vi "Reset SigGen.vi"(8 "error in (no error)":errorcluster, 11 "VISA Refnum in":refnum<visa-resource-name>) -> (0 "error out":errorcluster, 3 "VISA Refnum out":refnum<visa-resource-name>)   [LabVIEW 2015]
uses:
  <instrlib>/Agilent PSG MXG Series/Agilent PSG MXG Series.lvlib
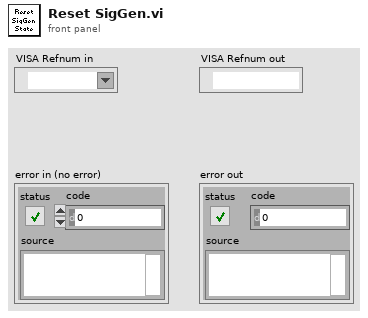
[diagram p1: front panel]
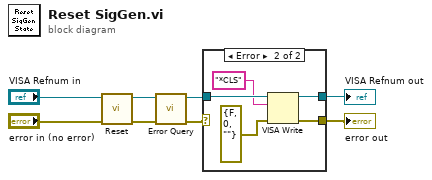
[diagram p0: block diagram]
diagram:
  n1 = call <instrlib>:"Reset.vi"("error in (no error)"="error in (no error)", "VISA resource name"="VISA Refnum in") -> ("error out"=w6:errorcluster, "VISA resource name out"=w5:refnum<visa-resource-name>)  [unwired: 8 in]
  n2 = call <instrlib>:"Error Query.vi"("error in (no error)"=w6, "VISA resource name"=w5) -> ("error out"=w3:errorcluster, "VISA resource name out"=w4:refnum<visa-resource-name>)  [unwired: 6 in, 2 out]
  n3 = case shown="Error" w3 {
    selector: w3 -> [w10 _]
    tunnel: [w9 w15] -> w1
    tunnel: w4 -> [w9 w14]
    tunnel: [w10 w13] -> w2
    frame No Error {
    }
    frame Error {
      n4 = VISA Write(VISA resource name=w14, write buffer="*CLS", error in (no error)=errorcluster {"status"=FALSE, "code"=0, "source"=""}) -> (VISA resource name out=w15:refnum<visa-resource-name>, error out=w13:errorcluster)  [unwired: 1 out]
    }
  }
  "VISA Refnum out" <- w1
  "error out" <- w2
